vi "Enum Camera Attributes.vi"(8 "error in (no error)":errorcluster, 9 "Visibility":T1=enum."Advanced", 10 "Root":string, 11 "IMAQdx Actor in":refnum<class "IMAQdx Actor.lvclass">) -> (0 "error out":errorcluster, 2 "Attirbutes Infos":T2[](array[typedef]), 3 "IMAQdx Actor out":refnum<class "IMAQdx Actor.lvclass">)   [LabVIEW 2020, in "IMAQdx Actor.lvlib" / "IMAQdx Actor.lvclass"]
uses:
  IMAQdx Actor.lvclass
  Camera Actor/Camera Actor/Camera Attribute Info.ctl
  <vilib>/vision/driver/IMAQdx.llb/IMAQdx Attribute Visibility.ctl
  IMAQdx Actor.lvclass/IMAQdx Actor.ctl
  <vilib>/vision/driver/NI_Vision_Acquisition_Software.lvlib
  <resource>/objmgr/imaqdx.rc
  Camera Actor/Camera Actor.lvlib
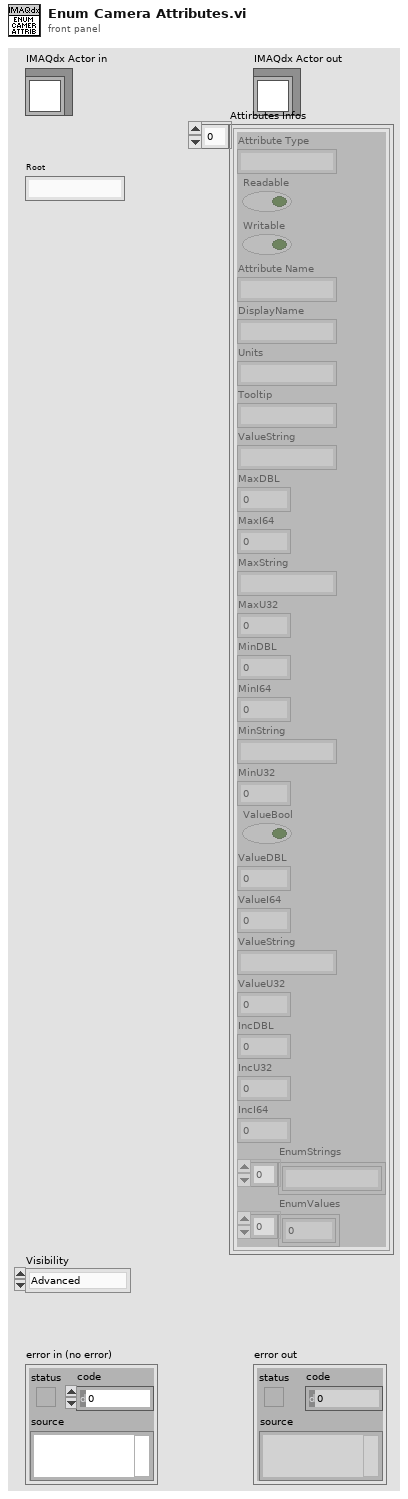
[diagram p1: front panel]
types:
  T1 = typedef "NI_Vision_Acquisition_Software.lvlib/IMAQdx Attribute Visibility.ctl" = enum32{"Simple", "Intermediate", "Advanced"}
  T2 = typedef "Camera Actor.lvlib/Camera Attribute Info.ctl" = cluster{"Attribute Type":string, "Readable":bool, "Writable":bool, "Attribute Name":string, "DisplayName":string, "Units":string, "Tooltip":string, "ValueString":string, "MaxDBL":dbl, "MaxI64":i64, "MaxString":string, "MaxU32":u32, "MinDBL":dbl, "MinI64":i64, "MinString":string, "MinU32":u32, "ValueBool":bool, "ValueDBL":dbl, "ValueI64 ":i64, "ValueString":string, "ValueU32":u32, "IncDBL":dbl, "IncU32":u32, "IncI64":i64, "EnumStrings":string[], "EnumValues":u32[]}
  T3 = typedef "IMAQdx.ctl" = refnum<k21>
  T4 = typedef "NI_Vision_Acquisition_Software.lvlib/IMAQdx Attribute Type.ctl" = enum32{"U32", "I64", "DBL", "String", "Enum", "Bool", "Command"}
  T5 = cluster{"Attribute Type":T4, "Readable":bool, "Writable":bool, "Attribute Name":string}[]
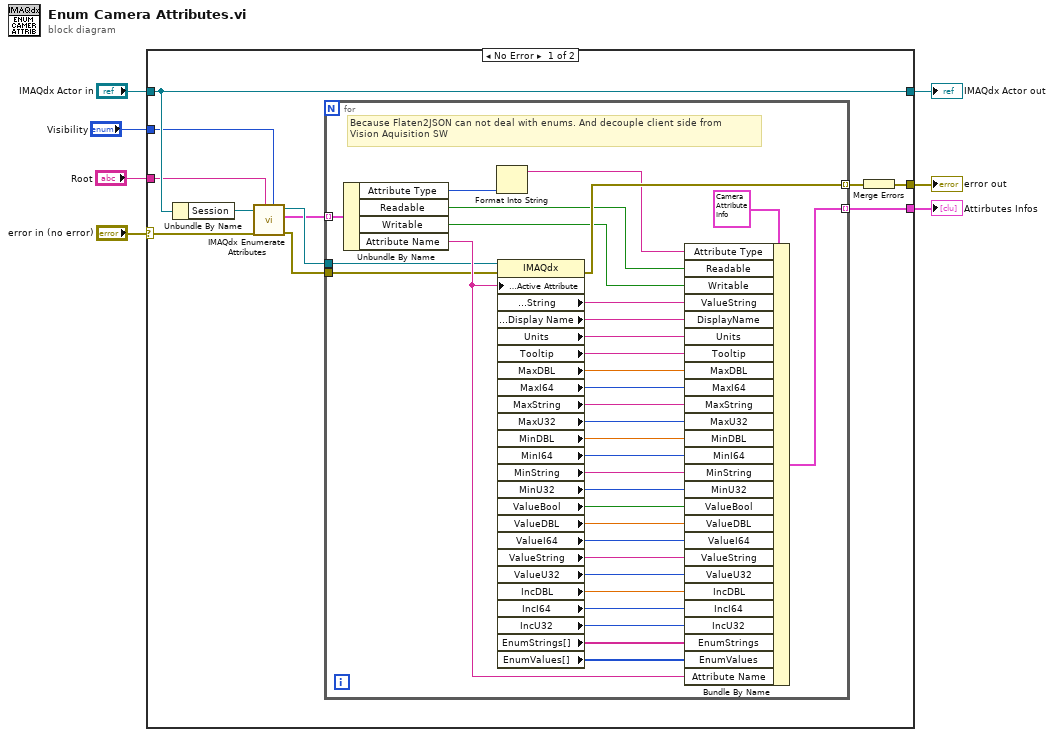
[diagram p0: block diagram]
diagram:
  n1 = case shown="No Error" "error in (no error)" {
    selector: "error in (no error)" -> [w16 w53]
    tunnel: [w12 w53] -> w6
    tunnel: [w18 w52] -> w4
    tunnel: "IMAQdx Actor in" -> [w18 w52]
    tunnel: [w11 _] -> w3
    tunnel: "Root" -> [w9 _]
    tunnel: "Visibility" -> [w8 _]
    frame No Error {
      n2 = Unbundle By Name(w18) -> ("Session"=w17:T3)
      n3 = call <vilib>:"IMAQdx Enumerate Attributes.vi"("Visibility"=w8, "Root"=w9, "error in"=w16, "Session In"=w17) -> ("error out"=w13:errorcluster, "Attribute Information Array"=w14:T5, "Session Out"=w15:T3)  [unwired: 5 in]
      n4 = for {
        tunnel: w15 -> [w49]
        tunnel: w14 -> [w48] mode=indexing
        tunnel: w13 -> [w42]
        tunnel: [w41] -> w11 mode=indexing
        tunnel: [w51] -> w10 mode=indexing
        # "Because Flaten2JSON can not deal with enums. And decouple client side from\nVision Aquisition SW"
        n5 = Unbundle By Name(w48) -> ("Attribute Type"=w46:T4, "Readable"=w30:bool, "Writable"=w29:bool, "Attribute Name"=w50:string)
        n6 = Format Into String(w46) -> (resulting string=w45:string)  [unwired: 3 in, 1 out]
        n7 = property class="IMAQdx"(reference=w49, error in=w42, "Camera Attributes:Active Attribute"=w50) -> (error out=w51:errorcluster, "Camera Attributes:Value:String"=w44:string, "Camera Attributes:Display Name"=w43:string, "Units"=w32:string, "Tooltip"=w31:string, "MaxDBL"=w40:dbl, "MaxI64"=w39:i64, "MaxString"=w38:string, "MaxU32"=w37:u32, "MinDBL"=w36:dbl, "MinI64"=w35:i64, "MinString"=w34:string, "MinU32"=w33:u32, "ValueBool"=w28:bool, "ValueDBL"=w27:dbl, "ValueI64"=w26:i64, "ValueString"=w25:string, "ValueU32"=w24:u32, "IncDBL"=w23:dbl, "IncI64"=w22:i64, "IncU32"=w21:u32, "EnumStrings[]"=w20:string[], "EnumValues[]"=w19:u32[])  [unwired: 1 out]
        n8 = Bundle By Name(cluster=T2 {"Attribute Type"="", "Readable"=FALSE, "Writable"=FALSE, "Attribute Name"="", "DisplayName"="", "Units"="", "Tooltip"="", "ValueString"="", "MaxDBL"=0.0, "MaxI64"=0, "MaxString"="", "MaxU32"=0, "MinDBL"=0.0, "MinI64"=0, "MinString"="", "MinU32"=0, "ValueBool"=FALSE, "ValueDBL"=0.0, "ValueI64 "=0, "ValueString"="", "ValueU32"=0, "IncDBL"=0.0, "IncU32"=0, "IncI64"=0, "EnumStrings"=[], "EnumValues"=[]} ("Attribute Information"), "Attribute Type"=w45, "Readable"=w30, "Writable"=w29, "ValueString"=w44, "DisplayName"=w43, "Units"=w32, "Tooltip"=w31, "MaxDBL"=w40, "MaxI64"=w39, "MaxString"=w38, "MaxU32"=w37, "MinDBL"=w36, "MinI64"=w35, "MinString"=w34, "MinU32"=w33, "ValueBool"=w28, "ValueDBL"=w27, "ValueI64"=w26, "ValueString"=w25, "ValueU32"=w24, "IncDBL"=w23, "IncI64"=w22, "IncU32"=w21, "EnumStrings"=w20, "EnumValues"=w19, "Attribute Name"=w50) -> (w41:T2)
      }
      n9 = Merge Errors(w10) -> (w12:errorcluster)
    }
    frame Error {
    }
  }
  "error out" <- w6
  "IMAQdx Actor out" <- w4
  "Attirbutes Infos" <- w3
